vi "ADO Connection Open by DSN path.vi"(6 "password":string, 7 "userID":string, 8 "error in (no error)":errorcluster caption="错误输入（无错误）", 9 "connection timeout (15)":i32=15, 10 "connection information":path, 11 "Database Connection 输入":refnum<class "Database Connection.lvclass"> caption="DNL_LabVIEW Object in") -> (0 "error out":errorcluster caption="错误输出", 3 "Database Connection 输出":refnum<class "Database Connection.lvclass"> caption="DNL_LabVIEW Object out")   [LabVIEW 2011, in "Database Connection.lvclass"]
uses:
  Database Connection.lvclass
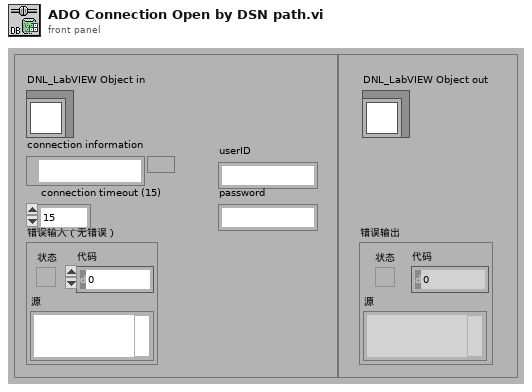
[diagram p1: front panel]
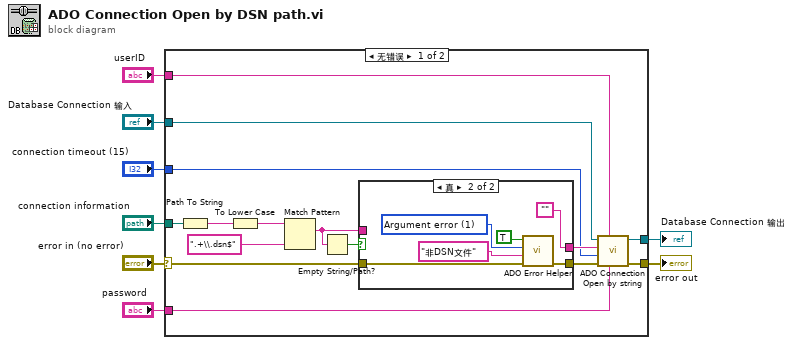
[diagram p0: block diagram]
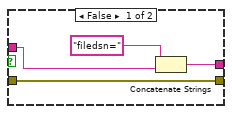
[diagram p2: hidden frame]
diagram:
  n1 = case shown="无错误" "error in (no error)" {
    selector: "error in (no error)" -> [w12 w35]
    tunnel: [w10 w35] -> w7
    tunnel: [w17 w34] -> w5
    tunnel: "Database Connection 输入" -> [w18 w34]
    tunnel: "connection information" -> [w21 _]
    tunnel: "userID" -> [w16 _]
    tunnel: "password" -> [w15 _]
    tunnel: "connection timeout (15)" -> [w13 _]
    frame No Error {
      n2 = Path To String(path=w21) -> (string=w22:string)
      n3 = To Lower Case(string=w22) -> (all lower case string=w23:string)
      n4 = Match Pattern(string=w23, regular expression=".+\\.dsn$") -> (match substring=w19:string)  [unwired: 4 out]
      n5 = Empty String/Path?(string/path=w19) -> (empty?=w20:bool)
      n6 = case shown="真" w20 {
        tunnel: w19 -> [w27 _]
        tunnel: [w26 ""] -> w14
        tunnel: w12 -> [w25 w30]
        tunnel: [w25 w29] -> w11
        frame False {
          n7 = Concatenate Strings("filedsn=" ("Substring"), w27) -> (w26:string)
        }
        frame True {
          w33 = 1 items=["No error", "Argument error", "Memory is full", "Out of zone", "End of file", "File already open", "Generic file I/O error", "File not found", "File permission error", "Disk is full", "Duplicate path", "Too many files open", "System feature not enabled", "Resource file not found", "Cannot add resource", "Resource not found", "Image not found", "Image memory error", "Pen does not exist", "Config type invalid", "Config token not found", "Config parse error", "Config memory error", "Bad external code format", "Bad external code offset", "External code not present", "Null window", "Destroy window error", "Null menu", "Print aborted", "Bad print record", "Print driver error", "Windows error during printing", "Memory error during printing", "Print dialog error", "Generic print error", "Invalid device refnum", "Device not found", "Device parameter error", "Device unit error", "Cannot open device", "Device call aborted", "Generic error", "Cancelled by user", "Object ID too low", "Object ID too high", "Object not in heap", "Unknown heap", "Unknown object (invalid DefProc)", "Unknown object (DefProc not in table)", "Message out of range", "Invalid (null) method", "Unknown message", "Manager call not supported", "Bad address", "Network operation in progress", "Network operation timed out", "Connection is busy", "Network attribute not supported", "Network error", "Address in use", "System out of memory", "Connection aborted", "Connection refused", "Not connected", "Already connected", "Connection closed", "Initialization error (interapplication manager)", "Bad occurrence", "Wait on unbound occurrence handler", "Occurrence queue overflow", "Datalog type conflict", "Unused", "Unrecognized type (interapplication manager)", "Memory corrupt", "Failed to make temporary DLL", "Old CIN version", "Drag socket not found", "Failed to load drop-object", "Failed to register OLE object", "Failed to release OLE object", "Format specifier type mismatch", "Unknown format specifier", "Too few format specifiers", "Too many format specifiers", "Scan failed", "Newer CIN version", "Error converting to variant", "Runtime menu error", "Password tampered", "Variant attribute not found", "Incompatible variant data type", "Event data is not available", "Event Store is not present", "Occurrence is not found", "Event Queue is not created", "Event info is not available", "Refnum passed is NULL", "Error retrieving Class GUID", "Error retrieving CoClass GUID", "Error retrieving TypeLib GUID.", "Bad built application magic bytes.", "Specific driver is different from the specific driver associated with the Logical Name.", "There is no session opened to the class driver.", "Max Error", "MAX - Error with config objects", "MAX - Error loading configuration", "MAX - Group not supported"]
          n8 = call "ADO Error Helper.vi"("Overriding error or warning"=w30, "source"="非DSN文件", "code"=w33, "status"=TRUE) -> ("error out"=w29:errorcluster)  [unwired: 7 in]
        }
      }
      n9 = call "ADO Connection Open by string.vi"("Password"=w15, "UserID"=w16, "error in (no error)"=w11, "connection timeout (15)"=w13, "ConnectionString"=w14, "Database Connection 输入"=w18) -> ("error out"=w10:errorcluster, "Database Connection 输出"=w17:refnum<class "Database Connection.lvclass">)  [unwired: 4 in]
    }
    frame Error {
    }
  }
  "error out" <- w7
  "Database Connection 输出" <- w5
